vi "ad find best range.vi"(6 "max":dbl, 7 "min":dbl, 8 "error in (no error)":errorcluster, 9 "range":i32, 10 "cha":i32, 11 "adh":i32) -> (0 "error out":errorcluster, 1 "range out":i32, 3 "function return":i32)   [LabVIEW 2021, in "libad4.lvlib"]
doc: "LIBAD4 fuction: ad_find_best_range (int32_t adh, int32_t cha, int32_t *range, double min, double max);\n\n\nUndocumented function."
uses:
  <userlib>/libad4/libad4.lvlib
  <userlib>/libad4/libad4.dll
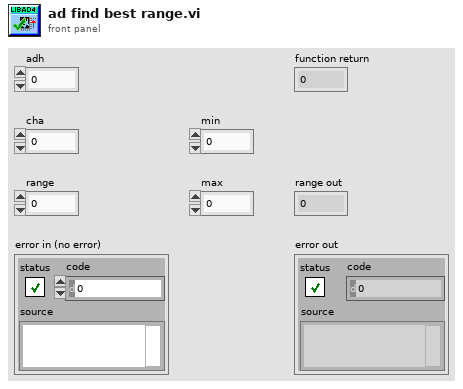
[diagram p1: front panel]
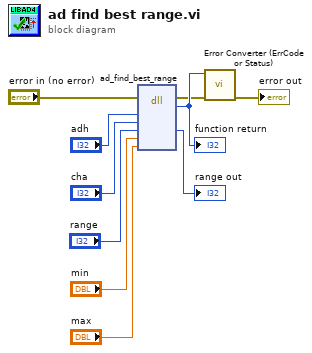
[diagram p0: block diagram]
diagram:
  n1 = dll-call lib="C:/Program Files/National Instruments/LabVIEW 2021/user.lib/libad4/libad4.*" fn="ad_find_best_range"(error in="error in (no error)", "adh"="adh", "cha"="cha", "range"="range", "min"="min", "max"="max") -> (error out=w2:errorcluster, w10:i32, "range"=→"range out":i32)  [unwired: 6 in, 1 out]
  "function return" <- w10
  n2 = call <userlib>:"Error Converter (ErrCode or Status).vi"("error in (no error)"=w2, "error code"=w10) -> ("error out"=→"error out":errorcluster)  [unwired: 9 in]
